vi "Replace VIs in Library (SubVI).vi"(8 "error out":errorcluster, 10 "Custom Device VIs":path[](array[path]), 11 "Custom Device Library":path) -> (0 "error out 2":errorcluster)   [LabVIEW 2010]
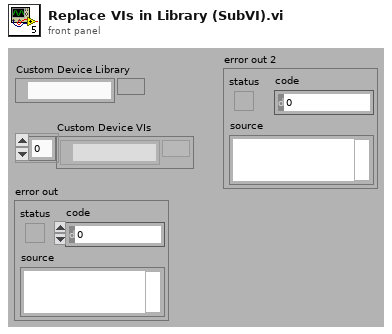
[diagram p1: front panel]
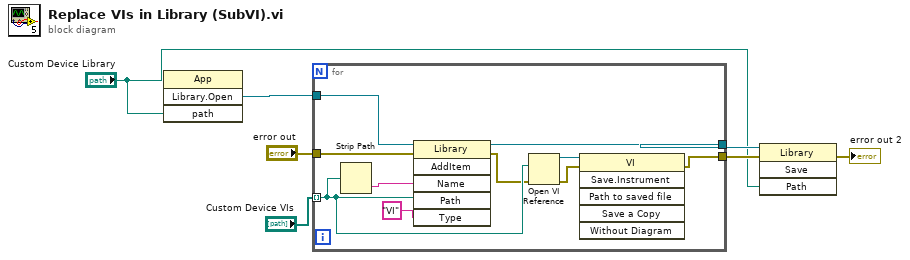
[diagram p0: block diagram]
diagram:
  n1 = invoke class="App" method="Library.Open"("path"="Custom Device Library") -> ("Open Library"=w2:refnum<vi>)  [unwired: 3 in, 3 out]
  n2 = for {
    tunnel: w2 -> [w17]
    tunnel: "error out" -> [w16]
    tunnel: "Custom Device VIs" -> [w12] mode=indexing
    tunnel: [w13] -> w6
    tunnel: [w8] -> w7
    n3 = Strip Path(path=w12) -> (name=w14:string)  [unwired: 1 out]
    n4 = invoke class="Library" method="AddItem"(reference=w17, error in=w16, "Name"=w14, "Path"=w12, "Type"="VI") -> (reference out=w13:refnum<vi>, error out=w9:errorcluster)  [unwired: 1 in, 4 out]
    n5 = Open VI Reference(vi path=w12, error in (no error)=w9) -> (vi reference=w11:refnum<vi>, error out=w10:errorcluster)  [unwired: 4 in]
    n6 = invoke class="VI" method="Save.Instrument"(reference=w11, error in=w10) -> (error out=w8:errorcluster)  [unwired: 4 in, 5 out]
  }
  n7 = invoke class="Library" method="Save"(reference=w6, error in=w7, "Path"="Custom Device Library") -> (error out=→"error out 2":errorcluster)  [unwired: 1 in, 3 out]
